vi "NewCore.vi"(8 "error in (no error)":errorcluster, 10 "ParamsArray":variant[](array[variant]), 11 "ChicagoStylePepperoniPizza":refnum<class "ChicagoStylePepperoniPizza.lvclass">) -> (0 "error out":errorcluster, 3 "ChicagoStylePepperoniPizza":refnum<class "ChicagoStylePepperoniPizza.lvclass">)   [LabVIEW 2020, in "FactoryMethod.lvlib" / "PizzaFactoryMethod.lvlib" / "ChicagoStylePepperoniPizza.lvclass"]
uses:
  ChicagoStylePepperoniPizza.lvclass
  Private/TypeDef/privateData.ctl
  ChicagoStylePepperoniPizza.lvclass/ChicagoStylePepperoniPizza.ctl
  Pizza/Pizza.lvclass
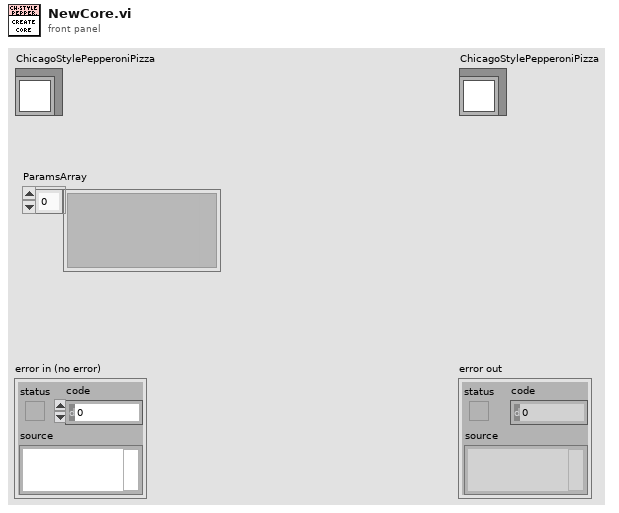
[diagram p1: front panel]
types:
  T1 = typedef "FactoryMethod.lvlib/PizzaFactoryMethod.lvlib/ChicagoStylePepperoniPizza.lvclass/privateData.ctl" = cluster{"Dummy":i32}
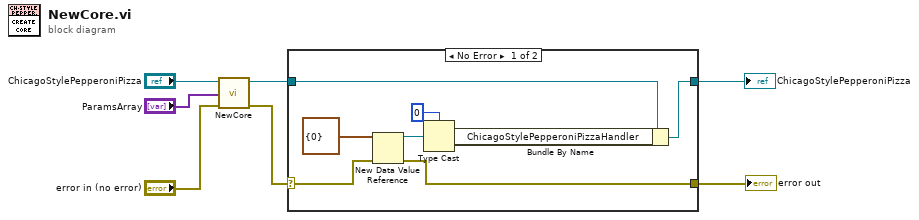
[diagram p0: block diagram]
diagram:
  n1 = call-parent "NewCore.vi"("error in"="error in (no error)", "ParamsArray"="ParamsArray", "Pizza"="ChicagoStylePepperoniPizza") -> ("error out"=w3:errorcluster, "Pizza"=w7:refnum<class "ChicagoStylePepperoniPizza.lvclass">)  [unwired: 7 in]
  n2 = case shown="No Error" w3 {
    selector: w3 -> [w8 w17]
    tunnel: [w10 w17] -> w5
    tunnel: [w12 w16] -> w6
    tunnel: w7 -> [w11 w16]
    frame No Error {
      n3 = New Data Value Reference(data value=T1 {"Dummy"=0} ("privateData"), error in=w8) -> (data value reference=w15:refnum<data-value>, error out=w10:errorcluster)
      n4 = Type Cast(type=u32 0, x=w15) -> (*(type *) &x=w13:u32)
      n5 = Bundle By Name(cluster=w11, "ChicagoStylePepperoniPizzaHandler"=w13) -> (w12:refnum<class "ChicagoStylePepperoniPizza.lvclass">)
    }
    frame Error {
    }
  }
  "error out" <- w5
  "ChicagoStylePepperoniPizza" <- w6
